vi "Handle error.vi"(8 "error in (no error)":errorcluster, 11 "RxTx in":refnum<class "RxTx.lvclass">) -> (0 "error out":errorcluster, 3 "RxTx out":refnum<class "RxTx.lvclass">)   [LabVIEW 2018, in "RxTx.lvclass"]
uses:
  RxTx.lvclass
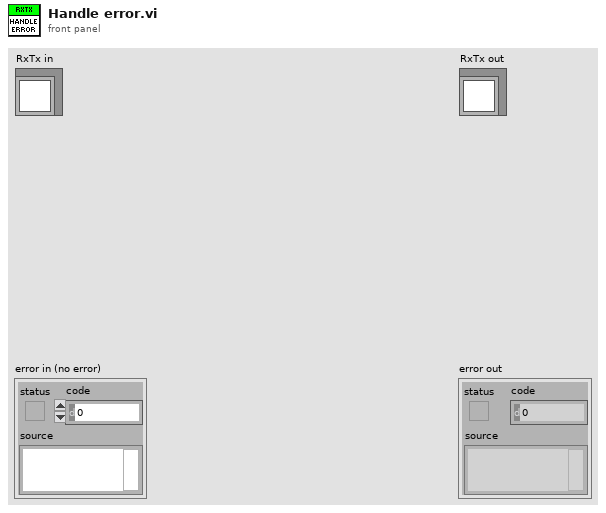
[diagram p1: front panel]
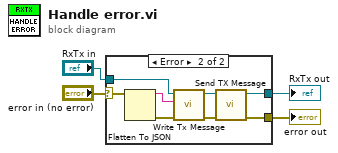
[diagram p0: block diagram]
diagram:
  n1 = case shown="Error" "error in (no error)" {
    selector: "error in (no error)" -> [w5 w7]
    tunnel: [w5 w9] -> w3
    tunnel: [w6 w10] -> w1
    tunnel: "RxTx in" -> [w6 w11]
    frame No Error {
    }
    frame Error {
      n2 = Flatten To JSON(anything=w7) -> (JSON string=w12:string, 11:w8:errorcluster)  [unwired: 2 in]
      n3 = call "Write Tx Message.vi"("error in (no error)"=w8, "Tx Message"=w12, "RxTx in"=w11) -> ("error out"=w13:errorcluster, "RxTx out"=w14:refnum<class "RxTx.lvclass">)  [unwired: 7 in]
      n4 = call "Send TX Message.vi"("error in (no error)"=w13, "RxTx in"=w14) -> ("error out"=w9:errorcluster, "RxTx out"=w10:refnum<class "RxTx.lvclass">)  [unwired: 8 in]
    }
  }
  "error out" <- w3
  "RxTx out" <- w1
